vi "Determine Warnings.vi"(1 "error in (no error)":errorcluster, 9 "MIn Temp":dbl, 10 "Max Temp":dbl, 11 "Current Temp":dbl) -> (0 "error out":errorcluster, 2 "Warning?":bool, 3 "Warning Text":string)   [LabVIEW 2014]
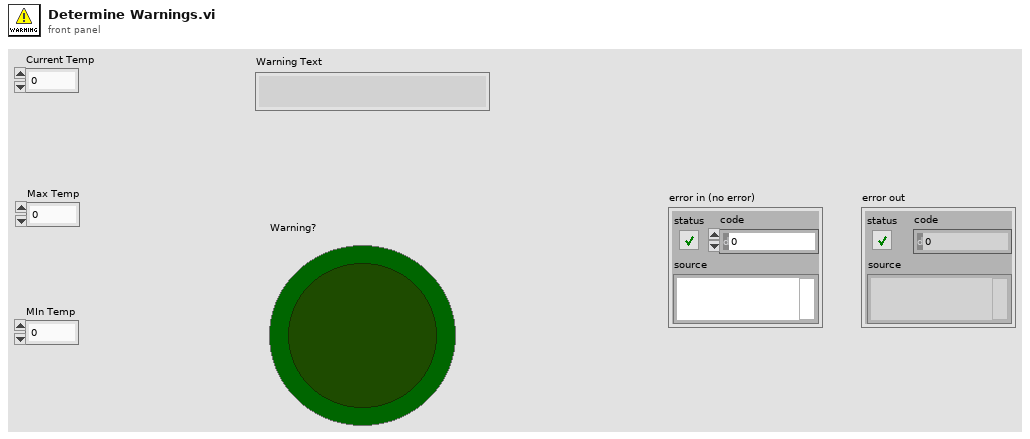
[diagram p1: front panel]
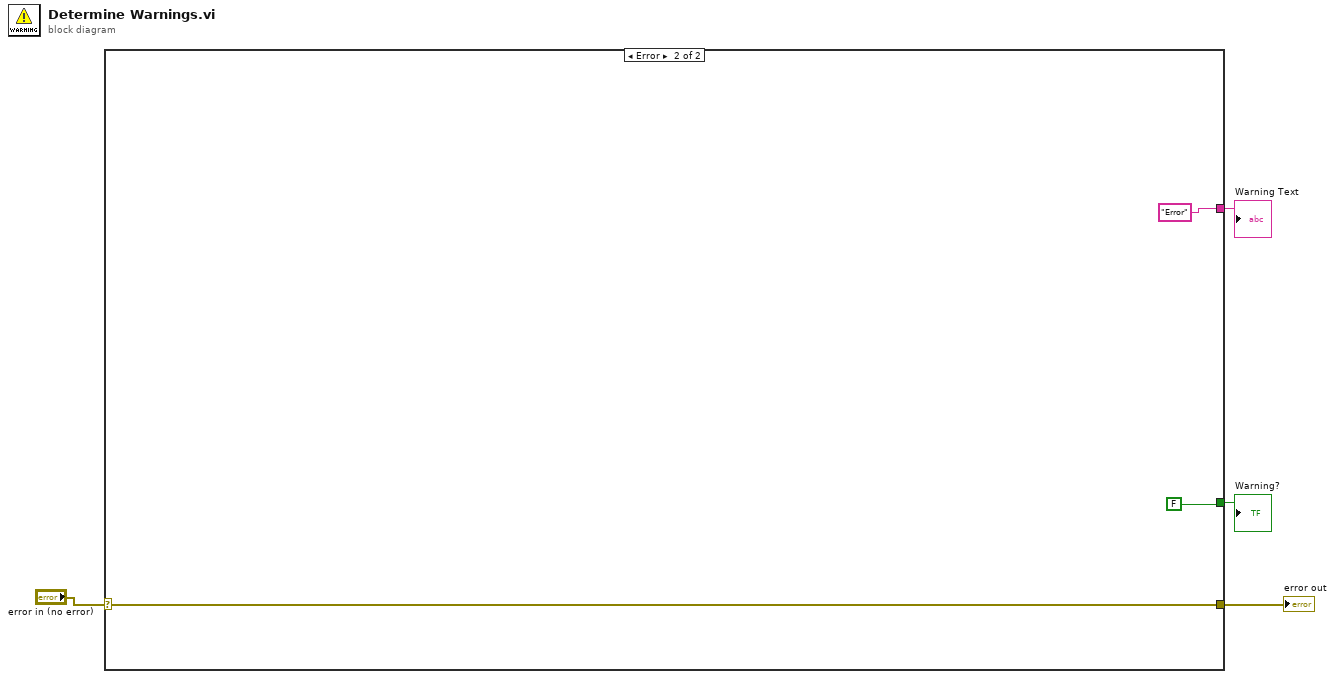
[diagram p0: block diagram]
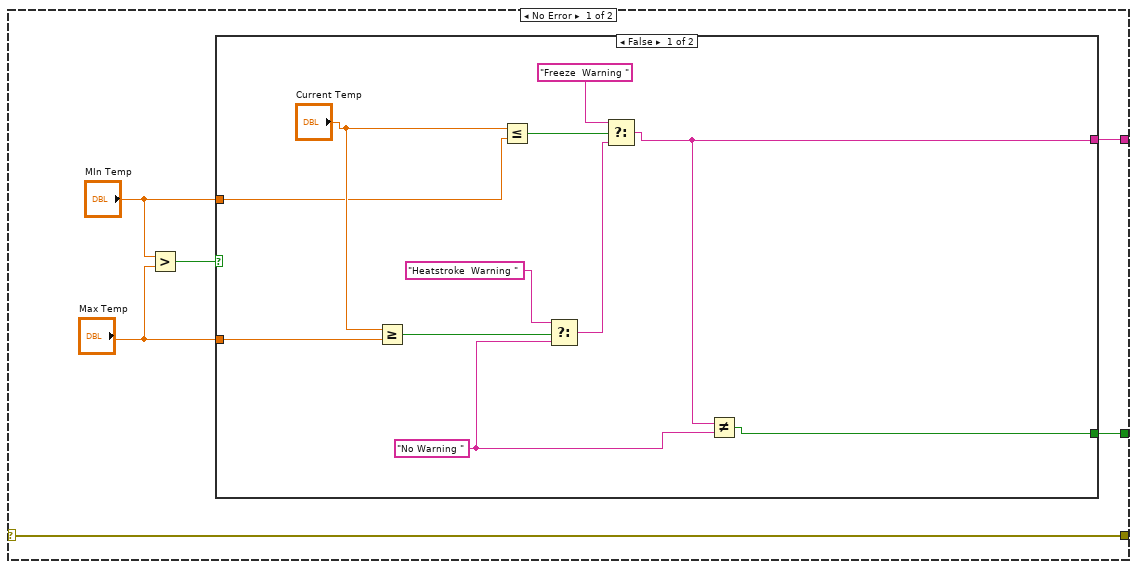
[diagram p2: hidden frame]
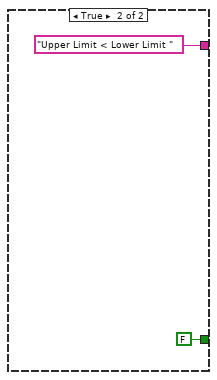
[diagram p3: hidden frame]
diagram:
  n1 = case shown="Error" "error in (no error)" {
    selector: "error in (no error)" -> [w5 w26]
    tunnel: [w7 "Error" ("Warning Text")] -> w4
    tunnel: [w6 FALSE ("Warning?")] -> w3
    tunnel: [w5 w26] -> w1
    frame No Error {
      n2 = Greater?(x="MIn Temp", y="Max Temp") -> (0:w8:bool)
      n3 = case shown="False" w8 {
        tunnel: "Max Temp" -> [w21 _]
        tunnel: "MIn Temp" -> [w13 _]
        tunnel: [w12 "Upper Limit < Lower Limit "] -> w7
        tunnel: [w11 FALSE ("Warning?")] -> w6
        frame False {
          w15 = "No Warning " ("String")
          n4 = Greater Or Equal?(x="Current Temp", y=w21) -> (x >= y?=w20:bool)
          n5 = Less Or Equal?(x="Current Temp", y=w13) -> (x <= y?=w18:bool)
          n6 = Select(t="Heatstroke  Warning " ("String"), s=w20, f=w15) -> (s? t:f=w16:string)
          n7 = Select(t="Freeze  Warning " ("String"), s=w18, f=w16) -> (s? t:f=w12:string)
          n8 = Not Equal?(x=w12, y=w15) -> (x != y?=w11:bool)
        }
        frame True {
        }
      }
    }
    frame Error {
    }
  }
  "Warning Text" <- w4
  "Warning?" <- w3
  "error out" <- w1
